vi "Start All Entry.vi"(7 "Project In":refnum<class "Project.lvclass">, 8 "error in (no error)":errorcluster, 10 "Input Control":T1[](array[typedef]), 11 "Entry Panel in":refnum<vi>[](array[refnum])) -> (0 "error out":errorcluster, 2 "Input Entry VI Refnum":refnum<vi>[](array[refnum]), 3 "Entry Panel out":refnum<vi>[](array[refnum]))   [LabVIEW 2015, in "CallVIStep.lvclass"]
uses:
  CallVIStep.lvclass
  VI Input Control Typedef.ctl
  VI Input Type Typedef.ctl
  Project.lvclass
  Input Entry.vi
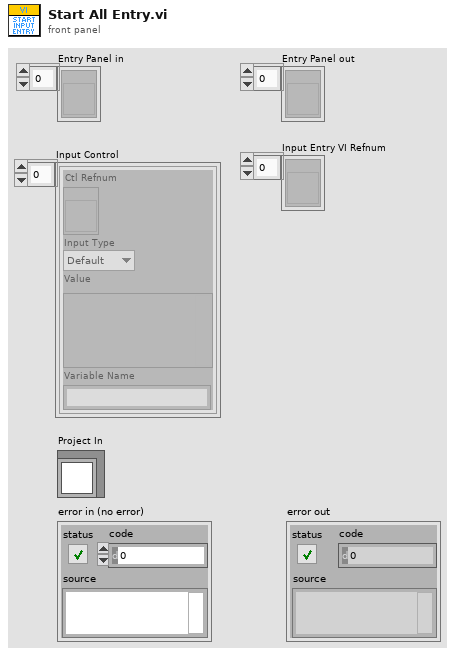
[diagram p1: front panel]
types:
  T1 = typedef "CallVIStep.lvclass/VI Input Control Typedef.ctl" = cluster{"Ctl Refnum":refnum<vi>, "Input Type":T2, "Value":variant, "Variable Name":string}
  T2 = typedef "CallVIStep.lvclass/VI Input Type Typedef.ctl" = enum16{"Default", "Value", "Variable"}
  T3 = enum32{"Invalid", "Standard", "Closed", "Hidden", "Minimized", "Maximized"}
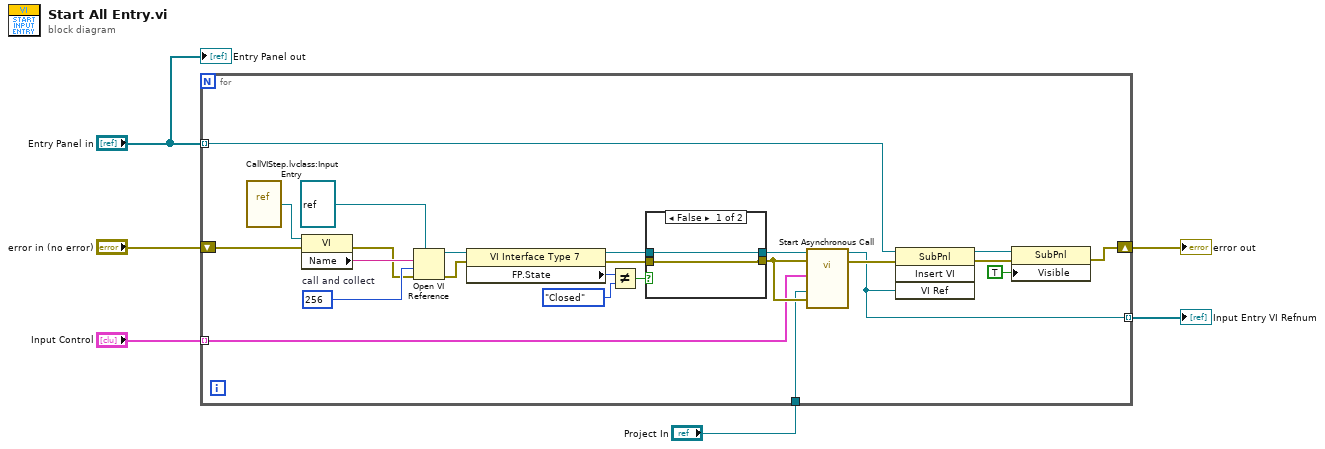
[diagram p0: block diagram]
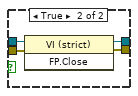
[diagram p2: hidden frame]
diagram:
  n1 = for {
    shift-right: [w9] -> w3
    shift-left: "error in (no error)" -> [w16]
    tunnel: "Input Control" -> [w12] mode=indexing
    tunnel: "Entry Panel in" -> [w14] mode=indexing
    tunnel: [w13] -> w2 mode=indexing
    tunnel: "Project In" -> [w7]
    w27 = 256  # call and collect
    n2 = vi-ref "CallVIStep.lvclass:Input Entry.vi"() -> (w30:refnum<vi>)
    n3 = property class="VI"(reference=w30, error in=w16) -> (error out=w26:errorcluster, "Name"=w28:string)  [unwired: 1 out]
    n4 = Open VI Reference(type specifier VI Refnum (for type only)=refnum<vi> refnum, vi path=w28, options=w27, error in (no error)=w26) -> (vi reference=w20:refnum<vi>, error out=w19:errorcluster)  [unwired: 2 in]
    n5 = property class="VI Interface Type 7"(reference=w20, error in=w19) -> (reference out=w24:refnum<vi>, error out=w25:errorcluster, "FP.State"=w21:T3)
    n6 = Not Equal?(x=w21, y=T3."Closed" ("Front Panel Window:State")) -> (x != y?=w23:bool)
    n7 = case shown="False" w23 {
      tunnel: w24 -> [w32 w36]
      tunnel: w25 -> [w31 w35]
      tunnel: [w32 w34] -> w18
      tunnel: [w31 w33] -> w17
      frame False {
      }
      frame True {
        n8 = invoke class="VI (strict)" method="FP.Close"(reference=w36, error in=w35) -> (reference out=w34:refnum<vi>, error out=w33:errorcluster)  [unwired: 1 in, 1 out]
      }
    }
    n9 = call-by-ref "Start Asynchronous Call"(reference=w18, error in=w17, 8:"error in (no error)"=w17, "Project In"=w7, "Input Control"=w12) -> (reference out=w13:refnum<vi>, error out=w15:errorcluster)  [unwired: 8 in, 1 out]
    n10 = invoke class="SubPnl" method="Insert VI"(reference=w14, error in=w15, "VI Ref"=w13) -> (reference out=w11:refnum<vi>, error out=w10:errorcluster)  [unwired: 1 in, 2 out]
    n11 = property class="SubPnl"(reference=w11, error in=w10, "Visible"=TRUE) -> (error out=w9:errorcluster)  [unwired: 1 out]
  }
  "error out" <- w3
  "Input Entry VI Refnum" <- w2
  "Entry Panel out" <- "Entry Panel in"
